vi "ARP Lookup.vi"(8 "error in (no error)":errorcluster, 10 "Address to ARP":u32 format="%08x", 11 "Address to ARP":string) -> (0 "error out":errorcluster, 2 "DMAC U64":u64 format="%.0x", 3 "DMAC String":string)   [LabVIEW 2021, in "Networking_CIF_U.lvlib"]
uses:
  Networking_CIF_U.lvlib
  Typedef/Errors.ctl
  Errors/Append Error Location.vi
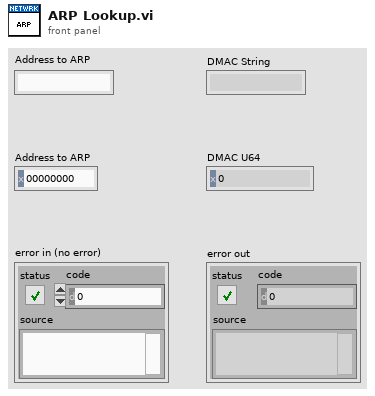
[diagram p1: front panel]
types:
  T1 = typedef "Networking_CIF_U.lvlib/Errors.ctl" = enum16{"Invalid IP Address", "No Subnet Match Found", "Error Finding Port", "No Ping Response", "Nettools Needed"}
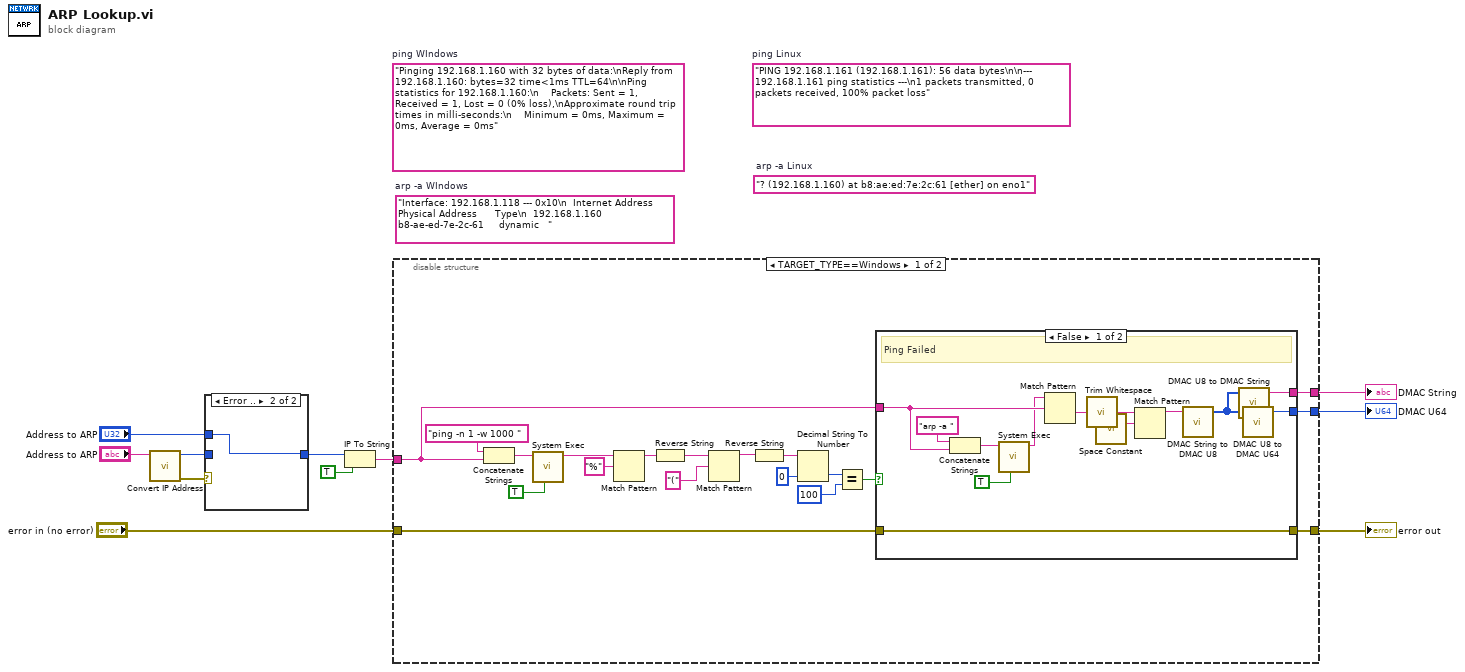
[diagram p0: block diagram]
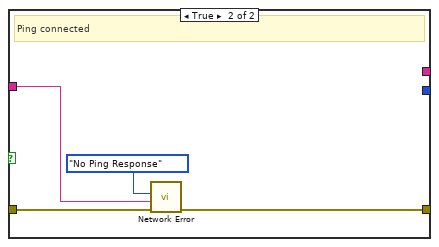
[diagram p3: hidden frame]
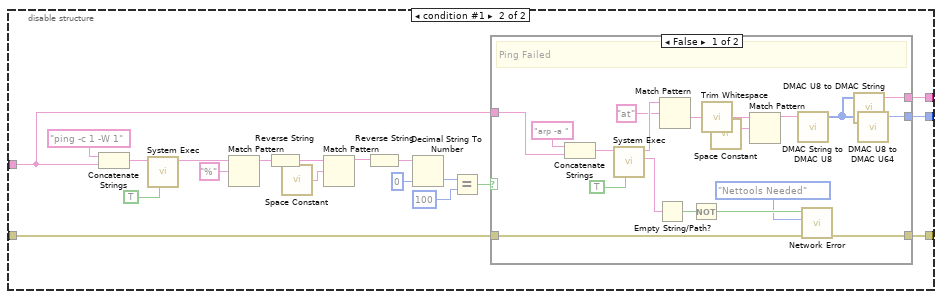
[diagram p4: hidden frame]
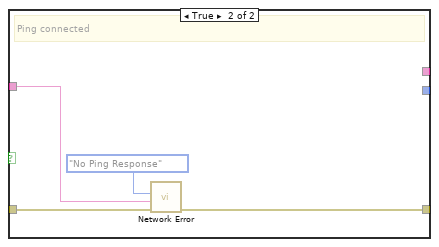
[diagram p5: hidden frame]
diagram:
  (unwired) "? (192.168.1.160) at b8:ae:ed:7e:2c:61 [ether] on eno1"  # arp -a Linux
  (unwired) "PING 192.168.1.161 (192.168.1.161): 56 data bytes\n\n--- 192.168.1.161 ping statistics ---\n1 packets transmitted, 0 packets received, 100% packet loss"  # ping Linux
  (unwired) "Pinging 192.168.1.160 with 32 bytes of data:\nReply from 192.168.1.160: bytes=32 time<1ms TTL=64\n\nPing statistics for 192.168.1.160:\n    Packets: Sent = 1, Received = 1, Lost = 0 (0% loss),\nApproximate round trip times in milli-seconds:\n    Minimum = 0ms, Maximum = 0ms, Average = 0ms"  # ping WIndows
  (unwired) "Interface: 192.168.1.118 --- 0x10\n  Internet Address      Physical Address      Type\n  192.168.1.160         b8-ae-ed-7e-2c-61     dynamic   "  # arp -a WIndows
  n1 = call "Convert IP Address.vi"("IP"="Address to ARP") -> ("error out"=w11:errorcluster, "net address"=w10:u32)  [unwired: 9 in]
  n2 = case shown="Error .." w11 {
    tunnel: w10 -> [w12 _]
    tunnel: [w12 w13] -> w6
    tunnel: "Address to ARP" -> [_ w13]
    frame No Error {
    }
    frame Error {
    }
  }
  n3 = IP To String(1:TRUE ("dot notation? (F)"), 2:w6) -> (0:w5:string)
  n4 = disable-structure shown="TARGET_TYPE==Windows" {
    disable-tunnel: w5 -> [w18 w52]
    disable-tunnel: [w17 w54] -> w4
    disable-tunnel: "error in (no error)" -> [w16 w51]
    disable-tunnel: [w15 w55] -> w2
    disable-tunnel: [w14 w53] -> w1
    frame condition #0 (active) {
      n5 = Concatenate Strings("ping -n 1 -w 1000 " ("command line"), w18) -> (w26:string)
      n6 = call <vilib>:"System Exec.vi"("run minimized? (F)"=TRUE, "command line"=w26) -> ("standard output"=w27:string)  [unwired: 6 in, 3 out]
      n7 = Match Pattern(string=w27, regular expression="%") -> (before substring=w28:string)  [unwired: 1 in, 3 out]
      n8 = Reverse String(1:w28) -> (0:w29:string)
      n9 = Match Pattern(string=w29, regular expression="(" ("command line")) -> (before substring=w30:string)  [unwired: 1 in, 3 out]
      n10 = Reverse String(1:w30) -> (0:w31:string)
      n11 = Decimal String To Number(string=w31, default (0L)=u8 0 ("default (0 I32)")) -> (number=w32:u8)  [unwired: 1 in, 1 out]
      n12 = Equal?(x=w32, y=u8 100) -> (x = y?=w19:bool)
      n13 = case shown="False" w19 {
        tunnel: w18 -> [w42 w48]
        tunnel: [w36 _] -> w17
        tunnel: w16 -> [w33 w49]
        tunnel: [w33 w46] -> w15
        tunnel: [w34 _] -> w14
        frame False {
          # "Ping Failed"
          n14 = Concatenate Strings("arp -a " ("command line"), w42) -> (w43:string)
          n15 = call <vilib>:"System Exec.vi"("run minimized? (F)"=TRUE, "command line"=w43) -> ("standard output"=w41:string)  [unwired: 6 in, 3 out]
          n16 = Match Pattern(string=w41, regular expression=w42) -> (after substring=w40:string)  [unwired: 1 in, 3 out]
          n17 = call <vilib>:"Trim Whitespace.vi"("string"=w40) -> ("trimmed string"=w39:string)  [unwired: 1 in]
          n18 = call <vilib>:"Space Constant.vi"() -> ("String"=w38:string)
          n19 = Match Pattern(string=w39, regular expression=w38) -> (before substring=w37:string)  [unwired: 1 in, 3 out]
          n20 = call "DMAC String to DMAC U8.vi"("DMAC String"=w37) -> ("DestinationMACAddress"=w35:u8[])  [unwired: 4 in]
          n21 = call "DMAC U8 to DMAC String.vi"("DestinationMACAddress"=w35) -> ("DMAC String"=w34:string)  [unwired: 4 in]
          n22 = call "DMAC U8 to DMAC U64.vi"("DestinationMACAddress"=w35) -> ("DMAC U64"=w36:u64)  [unwired: 4 in]
        }
        frame True {
          # "Ping connected"
          n23 = call "Network Error.vi"("error in (no error)"=w49, "String to Append"=w48, "Error"=Errors."No Ping Response") -> ("error out"=w46:errorcluster)  [unwired: 8 in]
        }
      }
    }
    frame condition #1 {
      n24 = Concatenate Strings("ping -c 1 -W 1" ("command line"), w52) -> (w62:string)
      n25 = call <vilib>:"System Exec.vi"("run minimized? (F)"=TRUE, "command line"=w62) -> ("standard output"=w63:string)  [unwired: 6 in, 3 out]
      n26 = Match Pattern(string=w63, regular expression="%") -> (before substring=w64:string)  [unwired: 1 in, 3 out]
      n27 = Reverse String(1:w64) -> (0:w65:string)
      n28 = call <vilib>:"Space Constant.vi"() -> ("String"=w50:string)
      n29 = Match Pattern(string=w65, regular expression=w50) -> (before substring=w66:string)  [unwired: 1 in, 3 out]
      n30 = Reverse String(1:w66) -> (0:w67:string)
      n31 = Decimal String To Number(string=w67, default (0L)=u8 0 ("default (0 I32)")) -> (number=w68:u8)  [unwired: 1 in, 1 out]
      n32 = Equal?(x=w68, y=u8 100) -> (x = y?=w56:bool)
      n33 = case shown="False" w56 {
        tunnel: w52 -> [w84 w90]
        tunnel: [w78 _] -> w54
        tunnel: w51 -> [w70 w91]
        tunnel: [w71 w88] -> w55
        tunnel: [w76 _] -> w53
        frame False {
          # "Ping Failed"
          n34 = Concatenate Strings("arp -a " ("command line"), w84) -> (w85:string)
          n35 = call <vilib>:"System Exec.vi"("run minimized? (F)"=TRUE, "command line"=w85) -> ("standard error"=w69:string, "standard output"=w83:string)  [unwired: 6 in, 2 out]
          n36 = Empty String/Path?(string/path=w69) -> (empty?=w74:bool)
          n37 = Match Pattern(string=w83, regular expression="at") -> (after substring=w82:string)  [unwired: 1 in, 3 out]
          n38 = Not(x=w74) -> (.not. x?=w73:bool)
          n39 = call <vilib>:"Trim Whitespace.vi"("string"=w82) -> ("trimmed string"=w81:string)  [unwired: 1 in]
          n40 = call <vilib>:"Space Constant.vi"() -> ("String"=w80:string)
          n41 = Match Pattern(string=w81, regular expression=w80) -> (before substring=w79:string)  [unwired: 1 in, 3 out]
          n42 = call "DMAC String to DMAC U8.vi"("DMAC String"=w79) -> ("DestinationMACAddress"=w77:u8[])  [unwired: 4 in]
          n43 = call "Network Error.vi"("error in (no error)"=w70, "Error"=Errors."Nettools Needed", "Insert Error"=w73) -> ("error out"=w71:errorcluster)  [unwired: 8 in]
          n44 = call "DMAC U8 to DMAC String.vi"("DestinationMACAddress"=w77) -> ("DMAC String"=w76:string)  [unwired: 4 in]
          n45 = call "DMAC U8 to DMAC U64.vi"("DestinationMACAddress"=w77) -> ("DMAC U64"=w78:u64)  [unwired: 4 in]
        }
        frame True {
          # "Ping connected"
          n46 = call "Network Error.vi"("error in (no error)"=w91, "String to Append"=w90, "Error"=Errors."No Ping Response") -> ("error out"=w88:errorcluster)  [unwired: 8 in]
        }
      }
    }
  }
  "DMAC U64" <- w4
  "error out" <- w2
  "DMAC String" <- w1
